vi "Configure DIAdem for Spartan.vi"(8 "error in (no error)":errorcluster) -> (0 "error out":errorcluster)   [LabVIEW 2011]
uses:
  <vilib>/Utility/sysdir.llb/System Directory Type.ctl
panel:
  out "PROBE:  New Config":string
  out "PROBE:  Original Config":string
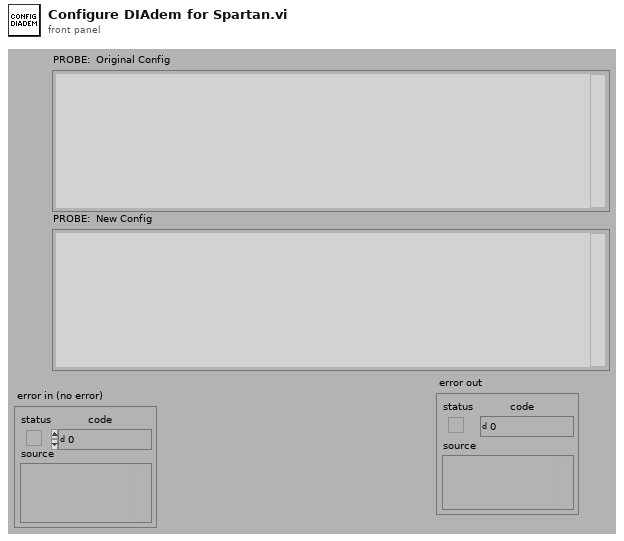
[diagram p1: front panel]
types:
  T1 = typedef "System Directory Type.ctl" = i32
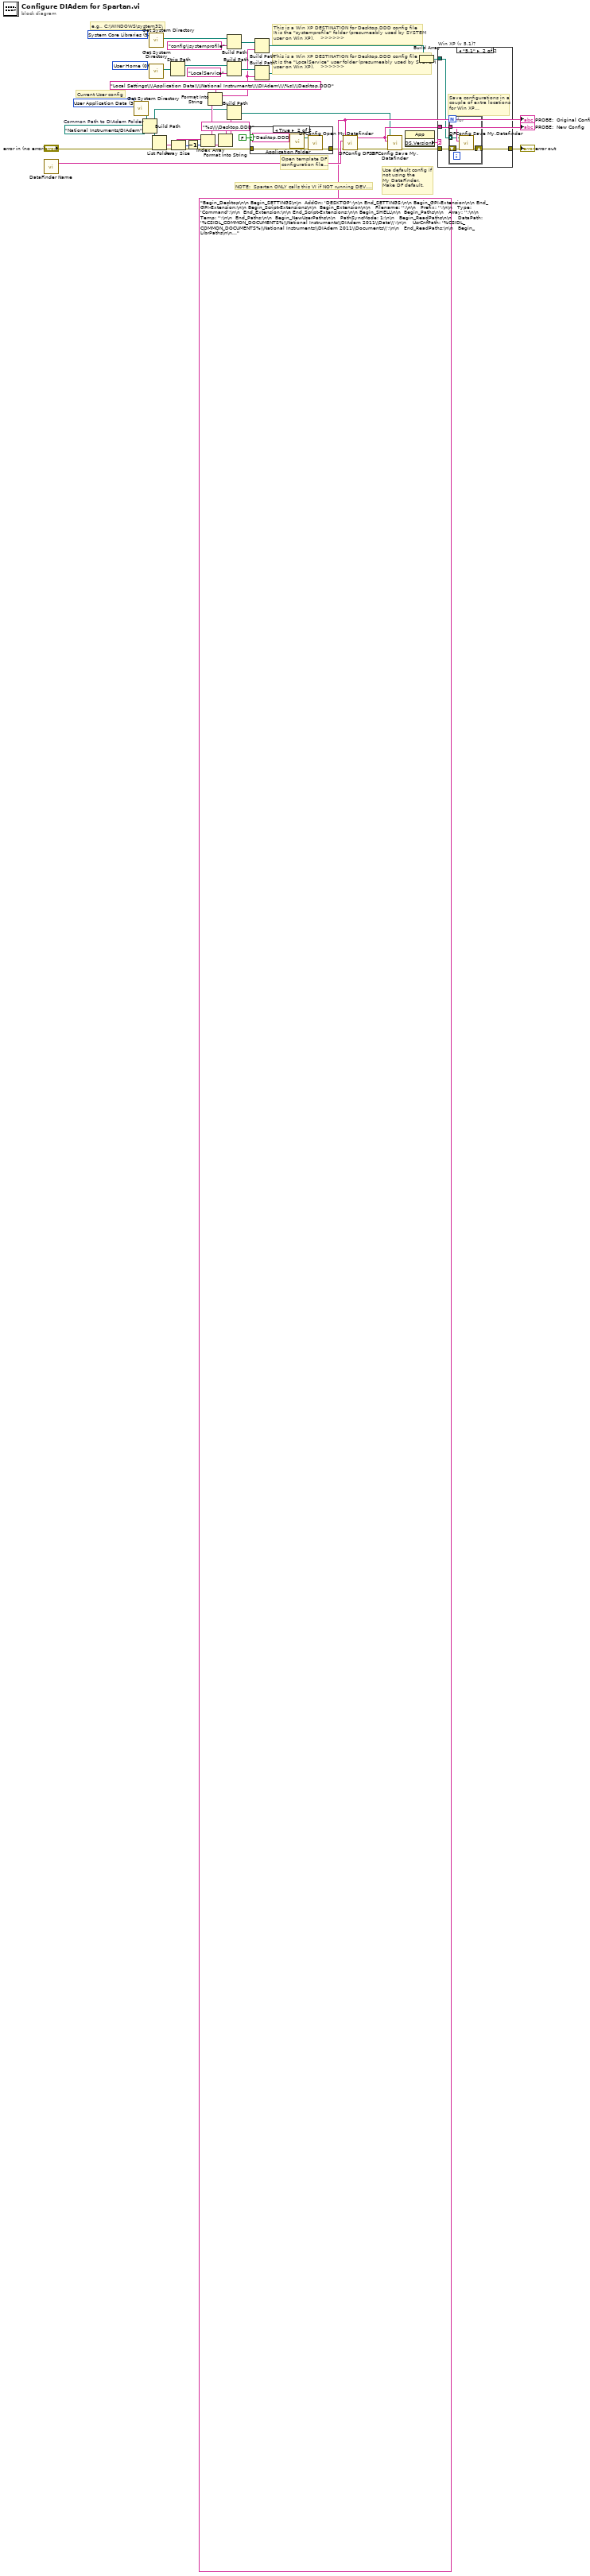
[diagram p0: block diagram]
diagram:
  w14 = path "National Instruments/DIAdem"  # Common Path to DIAdem Folder
  w16 = T1 3 items=["User Home", "User Desktop", "User Documents", "User Application Data", "User Preferences", "User Temporary", "Public Documents", "Public Application Data", "Public Preferences", "System Core Libraries", "System Installed Libraries", "Application Files", "Boot Volume Root"] ("system directory type")
  w26 = T1 0 items=["User Home", "User Desktop", "User Documents", "User Application Data", "User Preferences", "User Temporary", "Public Documents", "Public Application Data", "Public Preferences", "System Core Libraries", "System Installed Libraries", "Application Files", "Boot Volume Root"] ("system directory type")
  w30 = T1 9 items=["User Home", "User Desktop", "User Documents", "User Application Data", "User Preferences", "User Temporary", "Public Documents", "Public Application Data", "Public Preferences", "System Core Libraries", "System Installed Libraries", "Application Files", "Boot Volume Root"] ("system directory type")
  w32 = "Begin_Desktop\n\n Begin_SETTINGS\n\n  AddOn: 'DESKTOP';\n\n End_SETTINGS;\n\n Begin_GPI-Extension\n\n End_GPI-Extension;\n\n Begin_Script-Extensions\n\n  Begin_Extension\n\n   Filename: '';\n\n   Prefix: '';\n\n   Type: 'Command';\n\n  End_Extension;\n\n End_Script-Extensions;\n\n Begin_SHELL\n\n  Begin_Paths\n\n   Array: '';\n\n   Temp: '';\n\n  End_Paths;\n\n  Begin_NewUserPaths\n\n   PathSyncMode: 1;\n\n   Begin_ReadPaths\n\n    DataPath: '%CSIDL_COMMON_DOCUMENTS%\\National Instruments\\DIAdem 2011\\Data\\';\n\n    UsrCnfPath: '%CSIDL_COMMON_DOCUMENTS%\\National Instruments\\DIAdem 2011\\Documents\\';\n\n   End_ReadPaths;\n\n   Begin_LibrPaths\n\n    DataPath: 'libr\\Data\\';\n\n    UsrCnfPath: 'libr\\Documents\\';\n\n   End_LibrPaths;\n\n  End_NewUserPaths;\n\n  Begin_Universal\n\n   Sound: 'True';\n\n   TimeFormat: '#mm/dd/yyyy hh:nn:ss.ffff';\n\n   UseGlobTimeFormat: 'True';\n\n   LengthUnit: 'inch';\n\n   QuickInfoState: 'False';\n\n   ExitCheckChange: 'check';\n\n   FileCodingType: 'Unicode';\n\n   ExtendChnName: 'IndexName';\n\n   ExtEditorName: 'notepad.EXE';\n\n   WizReportIdxGen: 'False';\n\n   EqualBaseNaming: 'True';\n\n   SlashNoCtrlChar: 'True';\n\n   ToolInVBSSyntax: 'True';\n\n   UseNIFFT: 'True';\n\n   WriteResToChn: 'True';\n\n   CompResChnNaming: 'True';\n\n   TxtObjStdMode: 'True';\n\n   HideRegisterProp: 'True';\n\n   CompD3ScaleFrame: 'False';\n\n   UseNoValueOnCalcError: 'True';\n\n  End_Universal;\n\n  Begin_Textparams\n\n   FaceName: '';\n\n   Family: 0;\n\n   Charset: 0;\n\n   Size: 3;\n\n   Color: 'black';\n\n   Angle: 0;\n\n   Position: 'cent.';\n\n   Weight: 'False';\n\n   Italic: 'False';\n\n   Underline: 'False';\n\n   Strikeout: 'False';\n\n   Frame: 'False';\n\n   Clip: 'No';\n\n  End_Textparams;\n\n  Begin_LogFile\n\n   Size: 1000;\n\n   PartToReserve: 20;\n\n   Error: 'True';\n\n   Message: 'False';\n\n   Set: 'False';\n\n   Auto: 'False';\n\n   LogFileEditName: 'Notepad.exe';\n\n  End_LogFile;\n\n  Begin_Reserve\n\n   RAM: 24000;\n\n   VIR: 5120;\n\n   PAGE: 4096;\n\n  End_Reserve;\n\n  Begin_ExternalProgram\n\n   Name: '';\n\n   Parameter: '';\n\n  End_ExternalProgram;\n\n  Begin_Printer\n\n   Left: 0.5;\n\n   Top: 0.5;\n\n   Width: 10;\n\n   Orientation: 'landscape';\n\n   VirtualPrintMemory: 'False';\n\n   PrintTransparency: 'True';\n\n  End_Printer;\n\n  Begin_UserDefindedColors\n\n  End_UserDefindedColors;\n\n End_SHELL;\n\n Begin_DATA\n\n  Begin_Defaults\n\n   ASAMBrowserState: 'False';\n\n   File: 'EXAMPLE.TDM';\n\n   Begin_Paths\n\n   End_Paths;\n\n  End_Defaults;\n\n  Begin_Workspace\n\n   NaviInitMode: 'FixDataFinder';\n\n   NaviInitStore: 'My DataFinder';\n\n   NaviWfImport: 'WfChnOrigin';\n\n   NaviExportDataType: 'Auto binary';\n\n   NaviPropInheritance: 'None';\n\n   NaviPropNamingSchema: 'TypeNamePropertyName';\n\n   NaviPropInheritanceDF: 'None';\n\n   NaviBulkDataLoadingMode: 'BulkDataLoadingOnWriteAccess';\n\n  End_Workspace;\n\n  Begin_DataArea\n\n   HeaderEditSize: 1060;\n\n   ChnMaxDyn: 0;\n\n   UseDynDatabase: 'True';\n\n   ForceDynStorage: 'True';\n\n  End_DataArea;\n\n  Begin_OverWriteLoadPreSettings\n\n   Name: 'False';\n\n   Comment: 'True';\n\n   ChannelNamingMode: 'GroupUnique';\n\n  End_OverWriteLoadPreSettings;\n\n  Begin_SavePreSettings\n\n   SaveMode: 'Channel';\n\n   SaveType: 'Auto binary';\n\n   CheckImplizit: 'False';\n\n   CheckInteger: 'False';\n\n   ASCII-Separator: ',';\n\n   ASCII-Realformat: '';\n\n   ASCII-IntegerLength: 0;\n\n   FileCodingType: 'Unicode';\n\n  End_SavePreSettings;\n\n  Begin_LoadPreSettings\n\n   BlankToNoValue: 'False';\n\n  End_LoadPreSettings;\n\n End_DATA;\n\n Begin_AUTOSEQUENCE\n\n  Begin_Defaults\n\n   Begin_Paths\n\n   End_Paths;\n\n   AutoTeachLstPath: 'False';\n\n   AutoTeachChnMode: 'True';\n\n   NewDlgDefinition: 'True';\n\n   DlgGenerate: 'SUDEditor';\n\n   Workspace: '';\n\n   AutoTeachLstVar: 'True';\n\n  End_Defaults;\n\n End_AUTOSEQUENCE;\n\n Begin_VIEW\n\n  Begin_Defaults\n\n   File: 'EXAMPLE';\n\n   ViewDelMode: 'MarkedValNoValue';\n\n   ViewFitMode: 'linear';\n\n  End_Defaults;\n\n End_VIEW;\n\n Begin_ANALYSIS\n\n  Begin_Defaults\n\n   CalculationSet: 'EXAMPLE';\n\n  End_Defaults;\n\n End_ANALYSIS;\n\n Begin_GRAPH\n\n  Begin_Defaults\n\n   File: 'EXAMPLE';\n\n   Templat: 'Template';\n\n   MetaResolution: 10000;\n\n   UseTextAlign: 'True';\n\n   ObjHighlight: 'True';\n\n   RenderingMode: 'eAntialiasingStandard';\n\n  End_Defaults;\n\n End_GRAPH;\n\nEnd_Desktop;"
  # "Use default config if\nnot using the\nMy DataFinder.\nMake DF default."
  # "Open template DF\nconfiguration file..."
  # "This is a Win XP DESTINATION for Desktop.DDD config file\nIt is the \"LocalService\" user folder (presumeably used by SYSTEM\nuser on Win XP).    >>>>>>"
  # "e.g., C:\\WINDOWS\\system32\\"
  # "This is a Win XP DESTINATION for Desktop.DDD config file\nIt is the \"systemprofile\" folder (presumeably used by SYSTEM\nuser on Win XP).    >>>>>>"
  # "Current User config"
  # "NOTE:  Spartan ONLY calls this VI if NOT running DEV...."
  n1 = call "DataFinder Name.vi"() -> ("DataFinder Name"=w33:string)  [unwired: 3 in]
  n2 = call <vilib>:"Get System Directory.vi"("system directory type"=w16) -> ("system directory"=w15:path)  [unwired: 10 in]
  n3 = Build Path(base path=w15, name or relative path=w14) -> (appended path=w4:path)
  n4 = call <vilib>:"Get System Directory.vi"("system directory type"=w30) -> ("system directory"=w29:path)  [unwired: 10 in]
  n5 = call <vilib>:"Get System Directory.vi"("system directory type"=w26) -> ("system directory"=w25:path)  [unwired: 10 in]
  n6 = List Folder(path=w4, error in="error in (no error)") -> (folder names=w11:string[], error out=w10:errorcluster)  [unwired: 2 in, 2 out]
  n7 = Strip Path(path=w25) -> (stripped path=w13:path)  [unwired: 1 out]
  n8 = Array Size(array=w11) -> (size(s)=w12:i32)
  n9 = Decrement(x=w12) -> (x-1=w2:i32)
  n10 = Index Array(array=w11, index=w2) -> (element=w6:string)
  n11 = Format Into String(format string="Local Settings\\\\Application Data\\\\National Instruments\\\\DIAdem\\\\%s\\\\Desktop.DDD", w6) -> (resulting string=w8:string)  [unwired: 2 in, 1 out]
  n12 = Format Into String(format string="%s\\\\Desktop.DDD", w6) -> (resulting string=w5:string)  [unwired: 2 in, 1 out]
  n13 = Build Path(base path=w4, name or relative path=w5) -> (appended path=w3:path)
  n14 = Build Path(base path=w29, name or relative path="config\\systemprofile" ("Path")) -> (appended path=w27:path)
  n15 = Build Path(base path=w13, name or relative path="LocalService" ("Path")) -> (appended path=w23:path)
  n16 = case shown="True" FALSE {
    tunnel: [w37 w41] -> w31
    tunnel: w10 -> [w37 w38]
    frame False {
    }
    frame True {
      n17 = call "Application Folder.vi"("Relative Path (\"\" - Folder)"="Desktop.DDD") -> ("Application Folder"=w40:path)  [unwired: 2 in]
      n18 = call "DFConfig Open My.Datafinder.vi"("error in (no error)"=w38, "my.datafinder Path (empty)"=w40) -> ("error out"=w41:errorcluster)  [unwired: 9 out]
    }
  }
  n19 = Build Path(base path=w27, name or relative path=w8) -> (appended path=w22:path)
  n20 = Build Path(base path=w23, name or relative path=w8) -> (appended path=w21:path)
  n21 = call "DFConfig DFSE.vi"("error in (no error)"=w31, "DF Name"=w33, "Desktop.DDD In"=w32) -> ("error out"=w17:errorcluster, "Desktop.DDD Out"=w34:string)  [unwired: 7 in]
  "PROBE:  New Config" <- w34
  n22 = call "DFConfig Save My.Datafinder.vi"("error in (no error)"=w17, "my.datafinder (\"\")"=w34, "my.datafinder Path (empty)"=w3) -> ("error out"=w18:errorcluster)  [unwired: 8 out]
  n23 = property class="App"() -> ("OS.Version"=w19:string)  [unwired: 2 in, 2 out]
  n24 = Build Array(w22, w21) -> (w20:path[])
  n25 = case "Win XP (v 5.1)?" shown="\"5.1\"" w19 {
    tunnel: w18 -> [w42 w45]
    tunnel: [w42 w44] -> w35
    tunnel: w34 -> [_ w46]
    tunnel: w20 -> [_ w43]
    frame Default {
    }
    frame "5.1" {
      # "Save configurations in a\ncouple of extra locations\nfor Win XP..."
      n26 = for {
        tunnel: w46 -> [w50]
        tunnel: w43 -> [w49] mode=indexing
        shift-right: [w47] -> w44
        shift-left: w45 -> [w48]
        n27 = call "DFConfig Save My.Datafinder.vi"("error in (no error)"=w48, "my.datafinder (\"\")"=w50, "my.datafinder Path (empty)"=w49) -> ("error out"=w47:errorcluster)  [unwired: 8 out]
      }
    }
  }
  "error out" <- w35
  "PROBE:  Original Config" <- w32
